vi "Dequeue Logs Element.vi"(8 "Error In":errorcluster, 9 "Timeout":i32=-1, 11 "EventLog in":refnum<class "ErrorLog.lvclass">) -> (0 "Error Out":errorcluster, 1 "Timed out?":bool, 3 "EventLog out":refnum<class "ErrorLog.lvclass">)   [LabVIEW 2019, in "ErrorLog.lvlib" / "ErrorLog.lvclass"]
uses:
  ErrorLog.lvclass
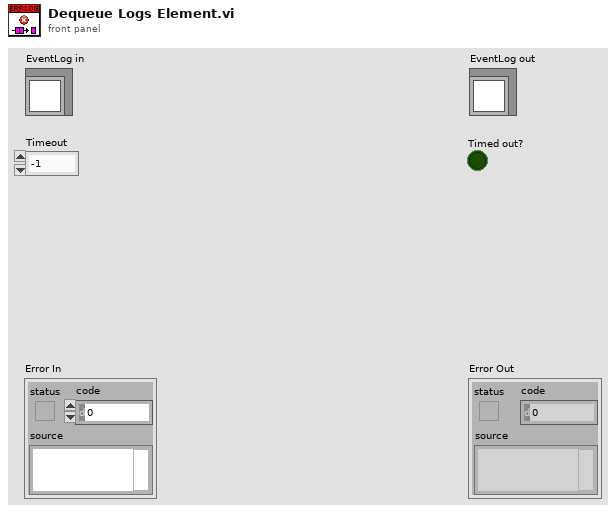
[diagram p1: front panel]
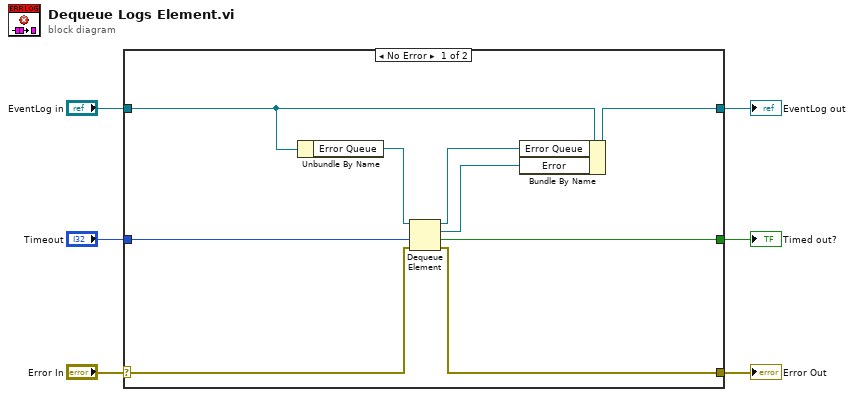
[diagram p0: block diagram]
diagram:
  n1 = case shown="No Error" "Error In" {
    selector: "Error In" -> [w14 w17]
    tunnel: [w13 w17] -> w6
    tunnel: [w12 w16] -> w4
    tunnel: "EventLog in" -> [w15 w16]
    tunnel: [w11 _] -> w5
    tunnel: "Timeout" -> [w10 _]
    frame No Error {
      n2 = Unbundle By Name(w15) -> ("Error Queue"=w9:refnum<queue>)
      n3 = Dequeue Element(queue=w9, timeout in ms (-1)=w10, error in (no error)=w14) -> (queue out=w7:refnum<queue>, element=w8:refnum<class "Error.lvclass">, timed out?=w11:bool, error out=w13:errorcluster)
      n4 = Bundle By Name(cluster=w15, "Error Queue"=w7, "Error"=w8) -> (w12:refnum<class "ErrorLog.lvclass">)
    }
    frame Error {
    }
  }
  "Error Out" <- w6
  "EventLog out" <- w4
  "Timed out?" <- w5
